vi "Write.vi"(8 "error in":errorcluster, 10 "Readings":digitalwaveform[](array[waveform]), 11 "Buffer Lossless Digital in":refnum<class "Buffer Lossless Digital.lvclass">) -> (0 "error out":errorcluster, 3 "Buffer Lossless Digital out":refnum<class "Buffer Lossless Digital.lvclass">)   [LabVIEW 2024, in "Buffer Lossless Digital.lvclass"]
uses:
  Buffer Lossless Digital.lvclass
  Buffer Lossless Digital.lvclass/Buffer Lossless Digital.ctl
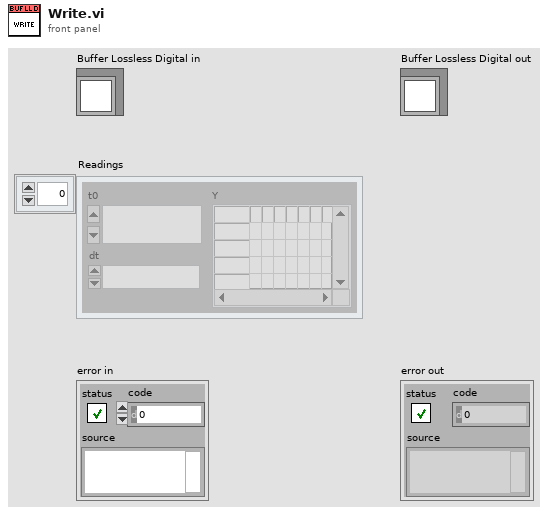
[diagram p1: front panel]
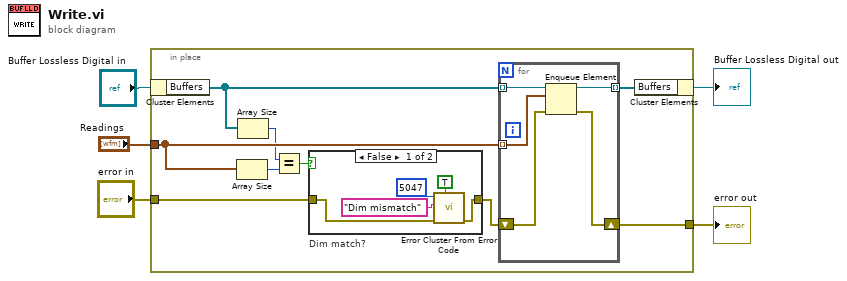
[diagram p0: block diagram]
diagram:
  n1 = in-place {
    in-place-border: "Readings" -> [w13]
    in-place-border: "error in" -> [w8]
    in-place-border: [w14] -> w1
    n2 = in-place-cluster #1("Buffer Lossless Digital in") -> ("Buffers"=w12:refnum<queue>[])
    n3 = Array Size(array=w13) -> (size(s)=w9:i32)
    n4 = Array Size(array=w12) -> (size(s)=w10:i32)
    n5 = Equal?(x=w10, y=w9) -> (x = y?=w11:bool)
    n6 = case "Dim match?" shown="False" w11 {
      tunnel: w8 -> [w19 w20]
      tunnel: [w18 w20] -> w7
      frame False {
        n7 = call <vilib>:"Error Cluster From Error Code.vi"("show call chain? (False)"=TRUE, "error in (no error)"=w19, "error message (\"\")"="Dim mismatch" ("error message (\"\")"), "error code (0)"=5047) -> ("error out"=w18:errorcluster)  [unwired: 5 in]
      }
      frame True {
      }
    }
    n8 = for {
      shift-right: [w22] -> w14
      shift-left: w7 -> [w23]
      tunnel: w13 -> [w24] mode=indexing
      tunnel: w12 -> [w25] mode=indexing
      tunnel: [w21] -> w6 mode=indexing
      n9 = Enqueue Element(queue=w25, element=w24, error in (no error)=w23) -> (queue out=w21:refnum<queue>, error out=w22:errorcluster)  [unwired: 1 in, 1 out]
    }
    n10 = in-place-cluster #1("Buffers"=w6) -> (→"Buffer Lossless Digital out":refnum<class "Buffer Lossless Digital.lvclass">)
  }
  "error out" <- w1
